vi "PID Block.vi"(7 "Deadband":dbl, 8 "From Shift":T1, 9 "Gains":cluster{"P":dbl, "I":dbl, "D":dbl}, 10 "Position":dbl format="%#_13g", 11 "Setpoint":dbl format="%#_13g") -> (0 "To Shift":T1, 2 "Tolerable?":bool, 3 "Output":dbl)   [LabVIEW 2014]
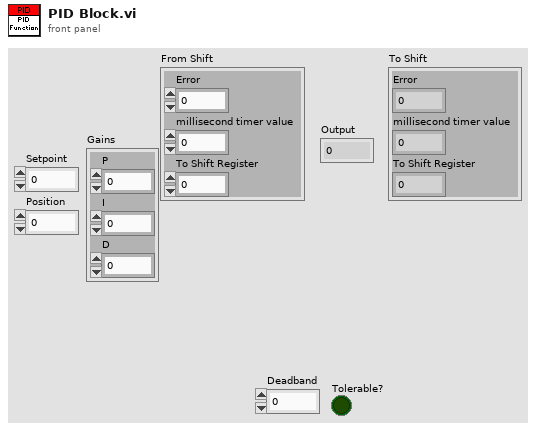
[diagram p1: front panel]
types:
  T1 = cluster{"Error":dbl, "millisecond timer value":u32, "To Shift Register":dbl}
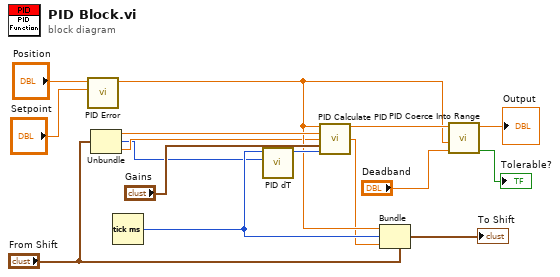
[diagram p0: block diagram]
diagram:
  n1 = call "PID Error.vi"("Setpoint"="Setpoint", "Position"="Position") -> ("Error"=w7:dbl)  [unwired: 9 in]
  n2 = Unbundle("From Shift") -> ("Error"=w8:dbl, "millisecond timer value"=w1:u32, "To Shift Register"=w3:dbl)
  n3 = Tick Count (ms)() -> (millisecond timer value=w12:u32)
  n4 = call "PID dT.vi"("Last Time"=w1, "Current Time"=w12) -> ("Change in Time"=w9:u32)  [unwired: 9 in]
  n5 = call "PID Calculate PID.vi"("Error"=w7, "Last Error"=w8, "From Shift Register"=w3, "Gains"="Gains", "Change in Time"=w9) -> ("Output"=w11:dbl, "To Shift Register"=w4:dbl)  [unwired: 9 in]
  n6 = Bundle(cluster="From Shift", "Error"=w7, "millisecond timer value"=w12, "To Shift Register"=w4) -> (→"To Shift":T1)
  n7 = call "PID Coerce Into Range.vi"("Deadband"="Deadband", "Error"=w7, "Output"=w11) -> ("Tolerable?"=→"Tolerable?":bool, "upper limit"=→"Output":dbl)  [unwired: 7 in]
